vi "test Basic Write Through Refnum.vi"(8 "error in (no error)":errorcluster, 11 "TestCase in":refnum<class "Refnum Tests.lvclass">) -> (0 "error out":errorcluster, 3 "TestCase out":refnum<class "Refnum Tests.lvclass">)   [LabVIEW 2024, in "Refnum Tests.lvclass"]
uses:
  Refnum Tests.lvclass
  <vilib>/Utility/file.llb/Application Directory.vi
  <vilib>/Utility/libraryn.llb/Check if File or Folder Exists.vi
  <vilib>/addons/_JKI Toolkits/VI Tester/TestCase.llb/TestCase.lvclass
  C:/Program Files/National Instruments/LabVIEW 2024/vi.lib/addons/_JKI Toolkits/VI Tester/TestCase.llb/TestCase.lvclass
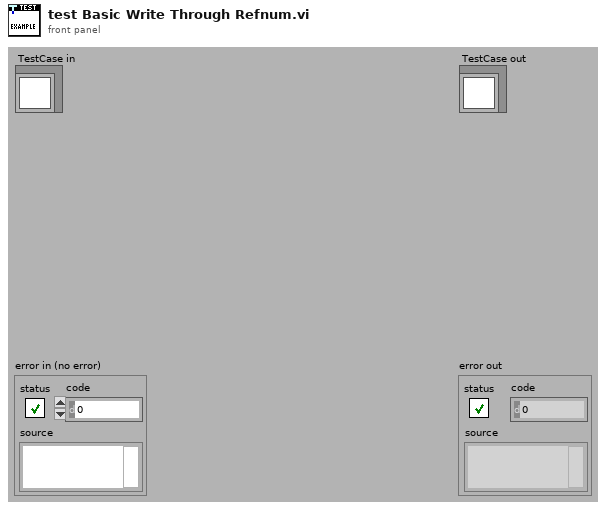
[diagram p1: front panel]
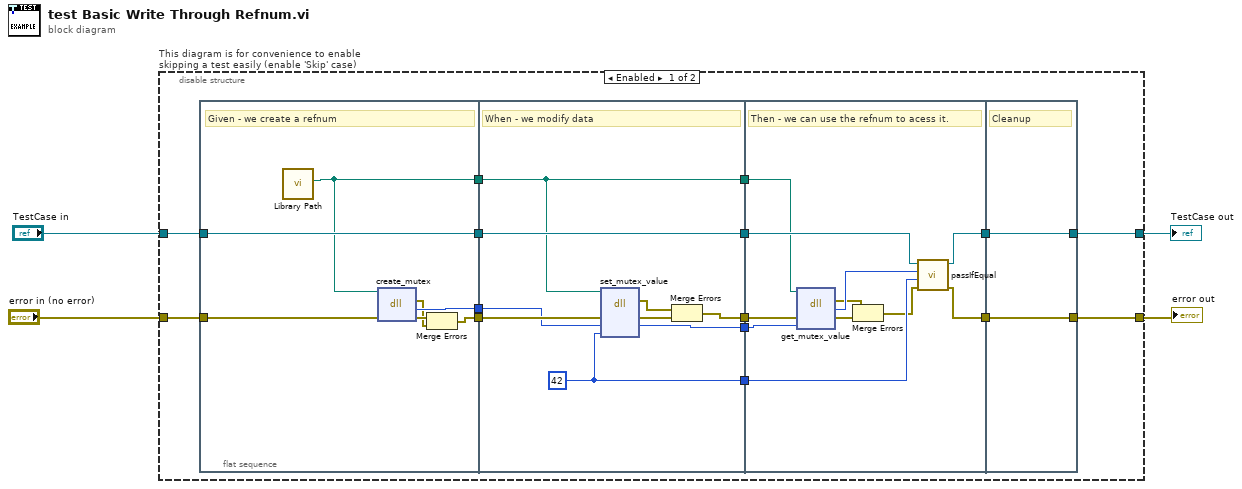
[diagram p0: block diagram]
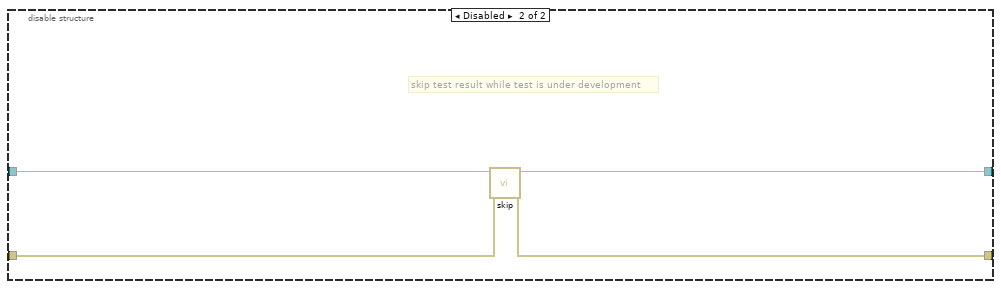
[diagram p2: hidden frame]
diagram:
  n1 = disable-structure "This diagram is for convenience to enable skipping a test easily (enable 'Skip' case)" shown="Enabled" {
    disable-tunnel: "TestCase in" -> [w12 w52]
    disable-tunnel: [w14 w50] -> w1
    disable-tunnel: [w13 w51] -> w3
    disable-tunnel: "error in (no error)" -> [w11 w49]
    frame Enabled {
      n2 = flat-sequence {
        tunnel: w11 -> [w24]
        tunnel: w12 -> [w26]
        tunnel: [w26] -> w19
        tunnel: [w25] -> w15
        tunnel: [w21] -> w10
        tunnel: [w22] -> w7
        tunnel: [w35] -> w18
        tunnel: w19 -> [w35]
        tunnel: w15 -> [w33]
        tunnel: w10 -> [w34]
        tunnel: [w33] -> w9
        tunnel: [w28] -> w8
        tunnel: w7 -> [w31]
        tunnel: [w30] -> w6
        tunnel: [w29] -> w5
        tunnel: [w45] -> w17
        tunnel: [w44] -> w16
        tunnel: w18 -> [w46]
        tunnel: w9 -> [w43]
        tunnel: w8 -> [w42]
        tunnel: w6 -> [w41]
        tunnel: w5 -> [w38]
        tunnel: [w47] -> w13
        tunnel: [w48] -> w14
        tunnel: w17 -> [w48]
        tunnel: w16 -> [w47]
        frame #0 {
          # "Given - we create a refnum"
          n3 = call "Library Path.vi"() -> ("Library Path"=w25:path)  [unwired: 11 in]
          n4 = dll-call lib="C:/Users/JamesMcNally/Documents/RustInterop/Rust-LabVIEW-Interop/target/debug/labview_test_library.dll" fn="create_mutex"(path in=w25, "err"=w24) -> (error out=w20:errorcluster, "return type"=w22:u32, "err"=w23:errorcluster)  [unwired: 2 in, 1 out]
          n5 = Merge Errors(w23, w20) -> (w21:errorcluster)
        }
        frame #1 {
          w29 = u8 42 ("value")
          # "When - we modify data"
          n6 = dll-call lib="C:/Users/JamesMcNally/Documents/RustInterop/Rust-LabVIEW-Interop/target/debug/labview_test_library.dll" fn="set_mutex_value"(path in=w33, "err"=w34, "refnum"=w31, "value"=w29) -> (error out=w27:errorcluster, "err"=w32:errorcluster, "refnum"=w30:u32)  [unwired: 4 in, 1 out]
          n7 = Merge Errors(w27, w32) -> (w28:errorcluster)
        }
        frame #2 {
          # "Then - we can use the refnum to acess it."
          n8 = dll-call lib="C:/Users/JamesMcNally/Documents/RustInterop/Rust-LabVIEW-Interop/target/debug/labview_test_library.dll" fn="get_mutex_value"(path in=w43, "err"=w42, "refnum"=w41) -> (error out=w36:errorcluster, "return type"=w40:u8, "err"=w39:errorcluster)  [unwired: 3 in, 1 out]
          n9 = Merge Errors(w36, w39) -> (w37:errorcluster)
          n10 = call-dynamic "passIfEqual.vi"("error in (no error)"=w37, "y"=w38, "x"=w40, "TestCase in"=w46) -> ("error out"=w44:errorcluster, "TestCase out"=w45:refnum<class "Refnum Tests.lvclass">)  [unwired: 6 in]
        }
        frame #3 {
          # "Cleanup"
        }
      }
    }
    frame Disabled {
      # "skip test result while test is under development"
      n11 = call <vilib>:"skip.vi"("error in (no error)"=w49, "TestCase in"=w52) -> ("error out"=w51:errorcluster, "TestCase out"=w50:refnum<class "Refnum Tests.lvclass">)  [unwired: 8 in]
    }
  }
  "error out" <- w3
  "TestCase out" <- w1
